vi "Self Test.vi"(8 "error in":errorcluster, 11 "SimELoad in":refnum<class "SimEload.lvclass">) -> (0 "error out":errorcluster, 2 "Self Test Passed?":bool, 3 "SimELoad out":refnum<class "SimEload.lvclass">)   [LabVIEW 2019, in "SimELoad.lvlib" / "SimEload.lvclass"]
uses:
  SimEload.lvclass
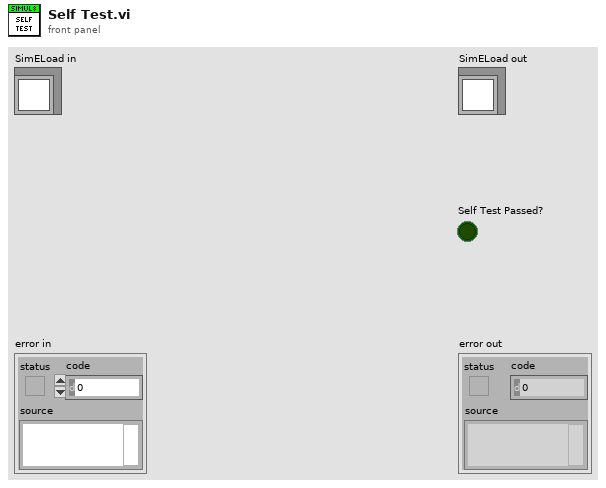
[diagram p1: front panel]
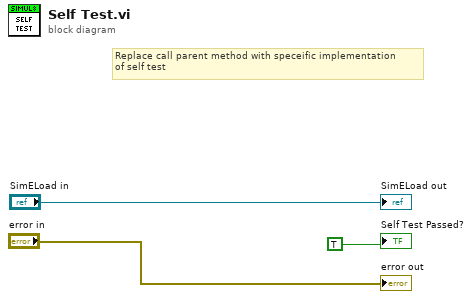
[diagram p0: block diagram]
diagram:
  # "Replace call parent method with speceific implementation\nof self test"
  "error out" <- "error in"
  "SimELoad out" <- "SimELoad in"
  "Self Test Passed?" <- TRUE
